vi "CIC_downsample5.vi"(8 "valid in":bool, 10 "din":fxp<+/-,20,16>) -> (0 "valid out":bool, 2 "dout":fxp<+/-,20,16>)   [LabVIEW 2013]
uses:
  <vilib>/rvi/FXPMathLib/FxpConvert/subVIs/nifxpmath_Convert_SimConfig.ctl
  <vilib>/fxp/LVFixedPointQuantizationPolicyTypeDef.ctl
  <vilib>/fxp/LVFixedPointOverflowPolicyTypeDef.ctl
  <vilib>/rvi/FXPMathLib/FxpConvert/simVIs/DllFxpConvertTemp_sub.vi
  <vilib>/rvi/IPIntegrationNode/IPINode_Utilities/niFpgaIPINodeSimCore.vi
  <vilib>/rvi/FXPMathLib/FxpConvert/XNode/nifxpmath_Convert.xnode
  <vilib>/rvi/XilinxIP/XIPIN_XNode/niFpgaXIPIN.xnode
  CIC_downsample5/CICdownsample5/CICdownsample5_F973C7B7B4784CD4B47288CBC28AFC1A.dll
  <vilib>/rvi/IPIntegrationNode/IPINode_Xnode/niFpgaIPINode.xnode
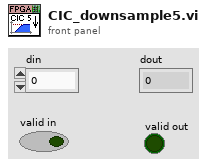
[diagram p1: front panel]
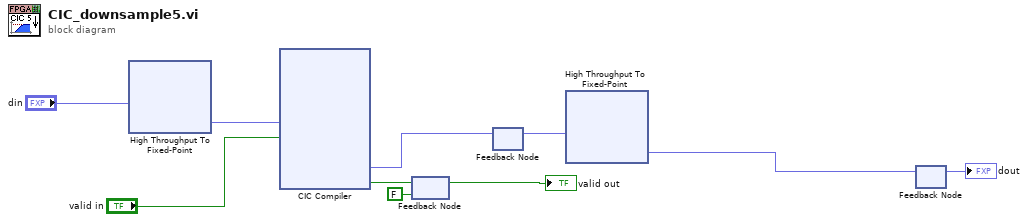
[diagram p0: block diagram]
diagram:
  n1 = xnode "High Throughput To Fixed-Point"("x"="din") -> ("y"=w2:fxp<+/-,24,20>)
  n2 = xnode ("CIC Compiler")("s_axis_data_tdata"=w2, "s_axis_data_tvalid"="valid in") -> ("m_axis_data_tdata"=w4:fxp<+/-,32,21>, "m_axis_data_tvalid"=w6:bool)  [unwired: 2 in, 1 out]
  n3 = feedback #1(FALSE ("rdy")) -> (→"valid out":bool)
  n4 = feedback-in #1(w6) -> ()
  n5 = feedback #2() -> (w1:fxp<+/-,32,21>)  [unwired: 1 in]
  n6 = feedback-in #2(w4) -> ()
  n7 = xnode "High Throughput To Fixed-Point"("x"=w1) -> ("y"=w3:fxp<+/-,20,16>)
  "dout" <- w3
  n8 = feedback #3() -> ()  [unwired: 2 in]
  n9 = feedback-in #3(w3) -> ()
